vi "Harvest OAuth Test.vi"() -> ()   [LabVIEW 2013]
uses:
  Oauth2.Harvest/Harvest Access Scopes.ctl
  OauthClient/OAuthClient.lvclass
  Oauth2/Oauth2.lvclass/Oauth2.ctl
  Oauth2/Read RefreshToken.vi
  Oauth2/Read ExpiresIn.vi
  Oauth2/Read Redirect URI.vi
  OAuthToken/Retrieve Element.vi
  Oauth2/Oauth2.lvclass
  <vilib>/LabVIEW Open Source Project/OpenURI/uri/URI.lvclass
  <vilib>/httpClient/LabVIEWHTTPClient.lvlib
  Oauth2.Harvest/Oauth2.Harvest.lvclass
panel:
  in  "Access Scope":T1={"all"=TRUE, "harvest:all"=FALSE, "forercast:all"=FALSE, "harvest:{accountID}"=FALSE, "forercast:{accountID}"=FALSE}
  out "REST API Error":errorcluster
  out "HTTP Response Headers":string
  out "Accounts":string
  out "Harvest Access Token":string
  out "Refresh Token":string
  out "Expires In":u32
  out "Redirect URI":string
  in  "Harvest API URL":string="https://id.getharvest.com/api/v2"
  out "Oauth Error":errorcluster
  in  "Query API Version":bool
  in  "Refresh":bool
  in  "Authorize":bool
  in  "Client Secret":string
  in  "Client ID":string
  # "Harvest Application API Access Example"
  # "G Open Source Project for LabVIEW\nhttps://github.com/LabVIEW-Open-Source/Oauth2"
  # "1- Get a Client ID and Client Secret from the application's admin. \n\n          * To access your own account, log into your site, create an application and set the access scope. \n          * This Oauth2.0 API uses the following redirect URL: http://localhost:58888/Oauth2/Redirect\n          * Record the client ID and client secret and fill in the fields below."
  # "3- Get an Access Token. You will be redirected your Harvest App's Authorization Server URI\n              * To authorize access, click on the \"Authorize App\" button.\n\n4- Once you have authenticated yourself, you will receive an access token.\n              * Use the \"Refresh Token\" button to request a fresh token\n                       OR\n              * Use the Access Token to query the Harvest API"
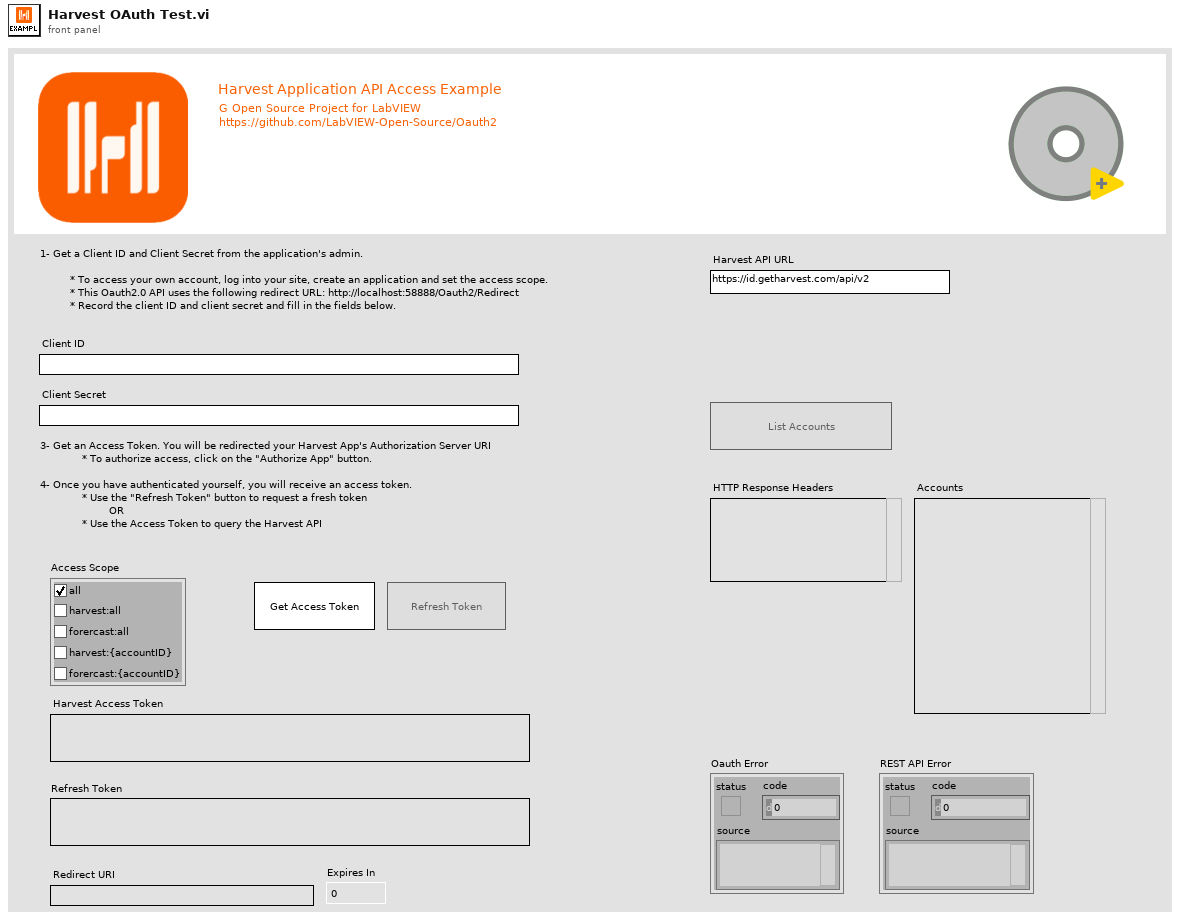
[diagram p1: front panel]
types:
  T1 = typedef "Oauth2.Harvest.lvclass/Harvest Access Scopes.ctl" = cluster{"all":bool, "harvest:all":bool, "forercast:all":bool, "harvest:{accountID}":bool, "forercast:{accountID}":bool}
  T2 = enum8{"Enabled", "Disabled", "Disabled and Grayed Out"}
  T3 = cluster{"Oauth2":refnum<class "Oauth2.Harvest.lvclass">, "Harvest API URL":string}
  T4 = typedef "LabVIEWHTTPClient.lvlib/ClientHandle.ctl" = refnum<k1>
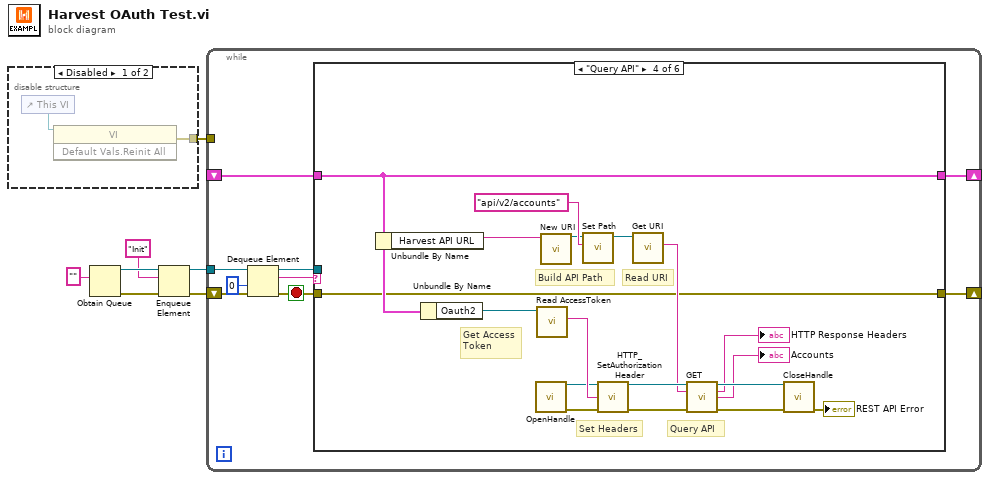
[diagram p0: block diagram]
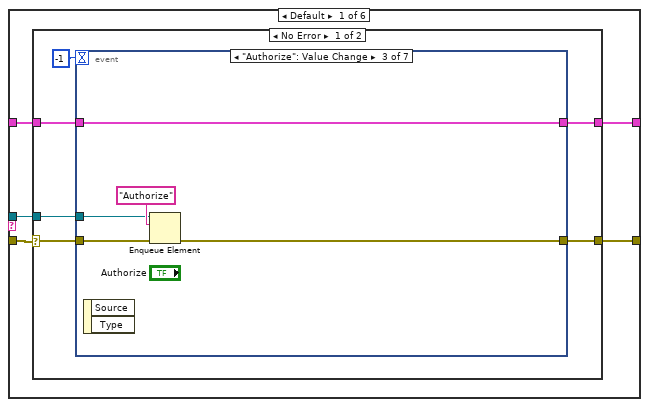
[diagram p3: hidden frame]
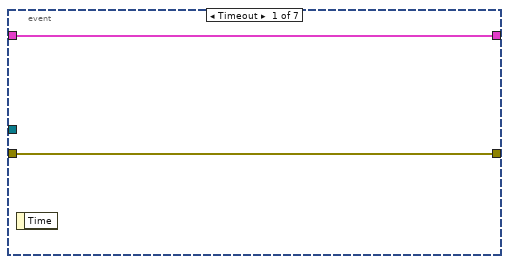
[diagram p4: hidden frame]
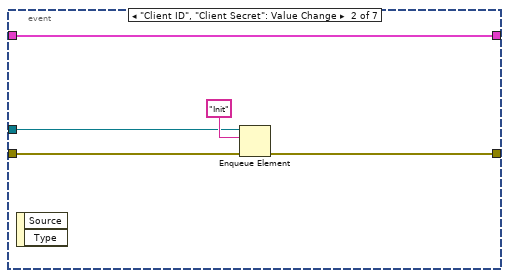
[diagram p5: hidden frame]
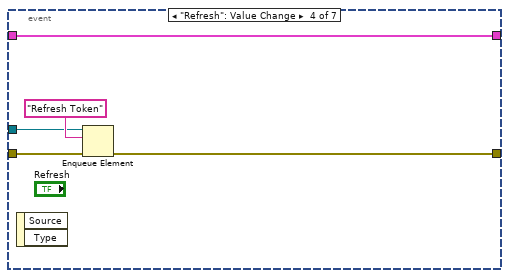
[diagram p6: hidden frame]
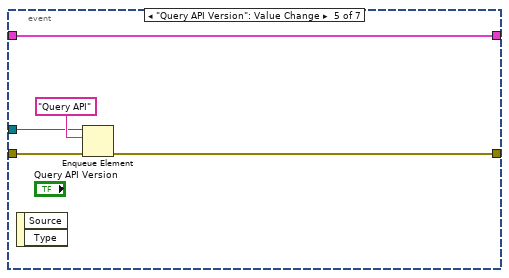
[diagram p7: hidden frame]
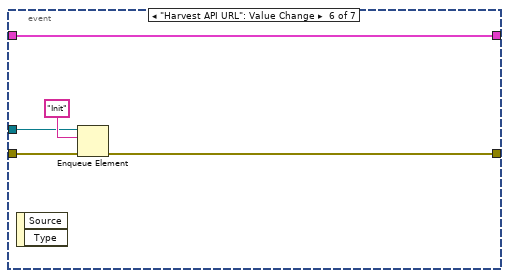
[diagram p8: hidden frame]
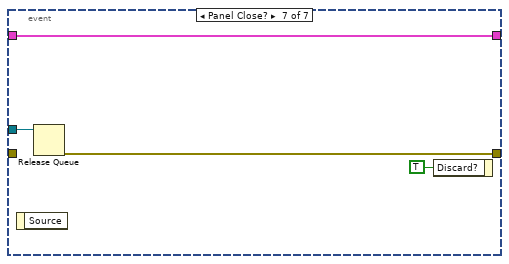
[diagram p9: hidden frame]
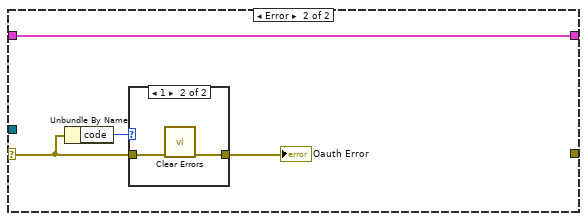
[diagram p10: hidden frame]
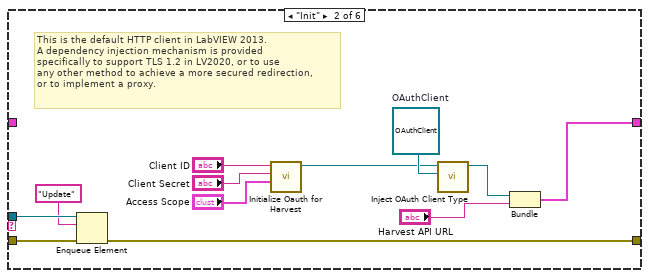
[diagram p12: hidden frame]
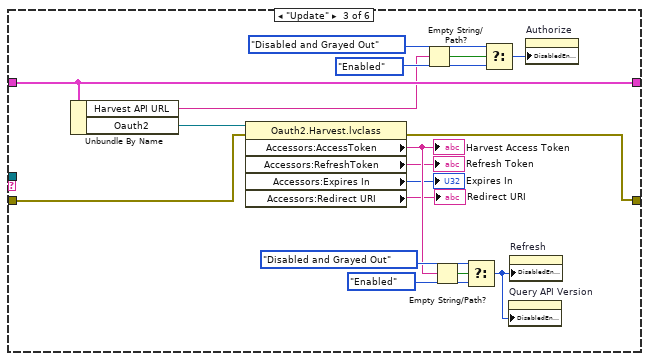
[diagram p13: hidden frame]
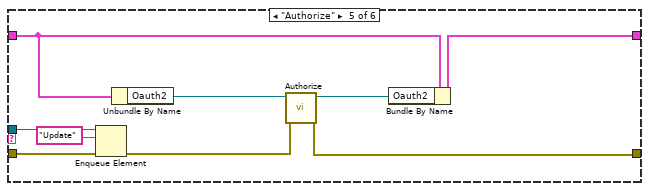
[diagram p14: hidden frame]
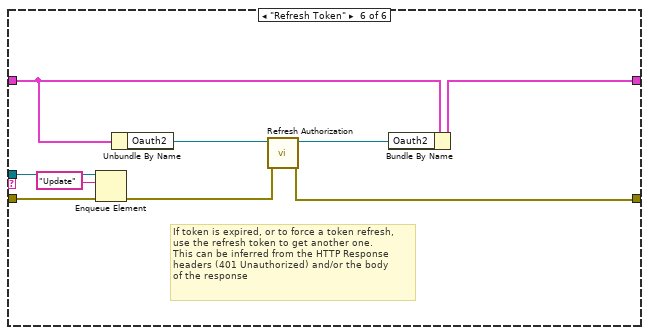
[diagram p15: hidden frame]
diagram:
  n1 = disable-structure shown="Disabled" {
    disable-tunnel: [w8 _] -> w1
    frame Disabled {
      n2 = control-ref of="This VI"() -> (w9:refnum<vi>)
      n3 = invoke class="VI" method="Default Vals.Reinit All"(reference=w9) -> (error out=w8:errorcluster)  [unwired: 2 in, 2 out]
    }
    frame Enabled {
    }
  }
  n4 = Obtain Queue(element data type="") -> (queue out=w4:refnum<queue>, error out=w6:errorcluster)  [unwired: 4 in, 1 out]
  n5 = Enqueue Element(queue=w4, element="Init", error in (no error)=w6) -> (queue out=w3:refnum<queue>, error out=w5:errorcluster)  [unwired: 1 in, 1 out]
  n6 = while {
    tunnel: w3 -> [w18]
    shift-right: [w13] -> _
    shift-left: _ -> [w12]
    shift-right: [w10] -> _
    shift-left: w5 -> [w14]
    tunnel: w1 -> [_]
    stop <- w11 stop-if-true
    n7 = Dequeue Element(queue=w18, timeout in ms (-1)=0, error in (no error)=w14) -> (queue out=w15:refnum<queue>, element=w16:string, error out=w11:errorcluster)  [unwired: 1 out]
    n8 = case shown="\"Query API\"" w16 {
      tunnel: w15 -> [w23 w78 _ _ w117 w129]
      tunnel: [w22 w79 w96 w111 w119 w131] -> w13
      tunnel: w12 -> [w21 _ w96 w111 w120 w132]
      tunnel: w11 -> [w20 w75 w86 w99 w116 w128]
      tunnel: [w19 w76 w85 w99 w122 w124] -> w10
      frame Default {
        n9 = case shown="No Error" w20 {
          selector: w20 -> [w24 w63]
          tunnel: w23 -> [w28 _]
          tunnel: [w27 w64] -> w22
          tunnel: w21 -> [w26 w64]
          tunnel: [w25 _] -> w19
          frame No Error {
            n10 = event shown="[2] \"Authorize\": Value Change" {
              selector: _ -> [_ _ _ _ _ _ _]
              dyn-events: _ -> [_ _ _ _ _ _ _]
              timeout: -1 -> [_ _ _ _ _ _ _]
              tunnel: w28 -> [_ w34 w40 w45 w50 w55 w60]
              tunnel: [w31 w36 w38 w43 w48 w53 w58] -> w27
              tunnel: w26 -> [w31 w36 w38 w43 w48 w53 w58]
              tunnel: [w30 w32 w37 w42 w47 w52 w57] -> w25
              tunnel: w24 -> [w30 w33 w39 w44 w49 w54 _]
              event Timeout {
                n11 = event-data() -> ()  [unwired: 1 in, 1 out]
              }
              event "Client ID", "Client Secret": Value Change {
                n12 = event-data() -> ()  [unwired: 1 in, 2 out]
                n13 = Enqueue Element(queue=w34, element="Init", error in (no error)=w33) -> (error out=w32:errorcluster)  [unwired: 1 in, 2 out]
              }
              event "Authorize": Value Change {
                n14 = event-data() -> ()  [unwired: 1 in, 2 out]
                n15 = Enqueue Element(queue=w40, element="Authorize", error in (no error)=w39) -> (error out=w37:errorcluster)  [unwired: 1 in, 2 out]
              }
              event "Refresh": Value Change {
                n16 = event-data() -> ()  [unwired: 1 in, 2 out]
                n17 = Enqueue Element(queue=w45, element="Refresh Token", error in (no error)=w44) -> (error out=w42:errorcluster)  [unwired: 1 in, 2 out]
              }
              event "Query API Version": Value Change {
                n18 = event-data() -> ()  [unwired: 1 in, 2 out]
                n19 = Enqueue Element(queue=w50, element="Query API", error in (no error)=w49) -> (error out=w47:errorcluster)  [unwired: 1 in, 2 out]
              }
              event "Harvest API URL": Value Change {
                n20 = event-data() -> ()  [unwired: 1 in, 2 out]
                n21 = Enqueue Element(queue=w55, element="Init", error in (no error)=w54) -> (error out=w52:errorcluster)  [unwired: 1 in, 2 out]
              }
              event Panel Close? {
                n22 = event-data() -> ()  [unwired: 1 in, 1 out]
                n23 = Release Queue(queue=w60) -> (error out=w57:errorcluster)  [unwired: 2 in, 2 out]
                n24 = event-data("Discard?"=TRUE) -> ()  [unwired: 1 in, 1 out]
              }
            }
          }
          frame Error {
            n25 = Unbundle By Name(w63) -> ("code"=w61:i32)
            n26 = case shown="1" w61 {
              tunnel: w63 -> [w65 w67]
              tunnel: [w65 w66] -> w62
              frame Default {
              }
              frame 1 {
                n27 = call <vilib>:"Clear Errors.vi"("error in (no error)"=w67) -> ("error out"=w66:errorcluster)  [unwired: 6 in]
              }
            }
            "Oauth Error" <- w62
          }
        }
      }
      frame "Init" {
        w74 = refnum<class "OAuthClient.lvclass"> refnum  # OAuthClient
        # "This is the default HTTP client in LabVIEW 2013.\nA dependency injection mechanism is provided\nspecifically to support TLS 1.2 in LV2020, or to use\nany other method to achieve a more secured redirection, \nor to implement a proxy."
        n28 = Enqueue Element(queue=w78, element="Update", error in (no error)=w75) -> (error out=w76:errorcluster)  [unwired: 1 in, 2 out]
        n29 = call "Initialize Oauth for Harvest.vi"("Harvest Access Scope"="Access Scope", "Client Secret"="Client Secret", "Client ID"="Client ID") -> ("Oauth2.Harvest"=w69:refnum<class "Oauth2.Harvest.lvclass">)  [unwired: 7 in, 1 out]
        n30 = call "Inject OAuth Client Type.vi"("OAuthClient"=w74, "Oauth2 in"=w69) -> ("Oauth2"=w73:refnum<class "Oauth2.Harvest.lvclass">)  [unwired: 9 in]
        n31 = Bundle("Oauth2"=w73, "Harvest API URL"="Harvest API URL") -> (w79:T3)  [unwired: 1 in]
      }
      frame "Update" {
        n32 = Unbundle By Name(w96) -> ("Harvest API URL"=w90:string, "Oauth2"=w91:refnum<class "Oauth2.Harvest.lvclass">)
        n33 = property class="Oauth2.Harvest.lvclass"(reference=w91, error in=w86) -> (error out=w85:errorcluster, "Accessors:AccessToken"=w84:string, "Accessors:RefreshToken"=→"Refresh Token":string, "Accessors:Expires In"=→"Expires In":u32, "Accessors:Redirect URI"=→"Redirect URI":string)  [unwired: 1 out]
        "Harvest Access Token" <- w84
        n34 = Empty String/Path?(string/path=w90) -> (empty?=w93:bool)
        n35 = Empty String/Path?(string/path=w84) -> (empty?=w89:bool)
        n36 = Select(t=T2."Disabled and Grayed Out" ("Disabled"), s=w89, f=T2."Enabled" ("Disabled")) -> (s? t:f=w80:T2)
        n37 = Select(t=T2."Disabled and Grayed Out" ("Disabled"), s=w93, f=T2."Enabled" ("Disabled")) -> (s? t:f=w92:T2)
        n38 = property on="Query API Version" class="Bool"("DisabledEnum"=w80) -> ()  [unwired: 2 in, 2 out]
        n39 = property on="Refresh" class="Bool"("DisabledEnum"=w80) -> ()  [unwired: 2 in, 2 out]
        n40 = property on="Authorize" class="Bool"("DisabledEnum"=w92) -> ()  [unwired: 2 in, 2 out]
      }
      frame "Query API" {
        # "Query API"
        # "Set Headers"
        # "Get Access\nToken"
        # "Read URI"
        # "Build API Path"
        n41 = Unbundle By Name(w111) -> ("Harvest API URL"=w107:string)
        n42 = Unbundle By Name(w111) -> ("Oauth2"=w112:refnum<class "Oauth2.Harvest.lvclass">)
        n43 = call <vilib>:"OpenHandle.vi"() -> ("client handle out"=w113:T4, "error out"=w104:errorcluster)  [unwired: 14 in]
        n44 = call "Read AccessToken.vi"("Oauth2 in"=w112) -> ("Access Token"=w114:string)  [unwired: 8 in, 2 out]
        n45 = call <vilib>:"New URI.vi"("URI"=w107) -> ("URI"=w108:refnum<class "URI.lvclass">)  [unwired: 9 in, 1 out]
        n46 = call <vilib>:"Set Path.vi"("path"="api/v2/accounts", "URI in"=w108) -> ("URI out"=w110:refnum<class "URI.lvclass">)  [unwired: 8 in, 1 out]
        n47 = call "HTTP_SetAuthorizationHeader.vi"("Client Handle"=w113, "Access Token"=w114, "error in (no error)"=w104) -> ("client handle dup"=w106:T4, "error out"=w103:errorcluster)  [unwired: 11 in]
        n48 = call <vilib>:"Get URI.vi"("URI in"=w110) -> ("URI String"=w105:string)  [unwired: 8 in, 2 out]
        n49 = call <vilib>:"GET.vi"("client handle"=w106, "url"=w105, "error in (no error)"=w103) -> ("client handle out"=w102:T4, "headers"=→"HTTP Response Headers":string, "body"=→"Accounts":string, "error out"=w101:errorcluster)  [unwired: 9 in]
        n50 = call <vilib>:"CloseHandle.vi"("client handle"=w102, "error in (no error)"=w101) -> ("error out"=→"REST API Error":errorcluster)  [unwired: 13 in]
      }
      frame "Authorize" {
        n51 = Enqueue Element(queue=w117, element="Update", error in (no error)=w116) -> (error out=w115:errorcluster)  [unwired: 1 in, 2 out]
        n52 = Unbundle By Name(w120) -> ("Oauth2"=w123:refnum<class "Oauth2.Harvest.lvclass">)
        n53 = call "Authorize.vi"("error in (no error)"=w115, "Oauth2 in"=w123) -> ("error out"=w122:errorcluster, "Oauth2 out"=w121:refnum<class "Oauth2.Harvest.lvclass">)  [unwired: 7 in, 1 out]
        n54 = Bundle By Name(cluster=w120, "Oauth2"=w121) -> (w119:T3)
      }
      frame "Refresh Token" {
        # "If token is expired, or to force a token refresh, \nuse the refresh token to get another one.\nThis can be inferred from the HTTP Response\nheaders (401 Unauthorized) and/or the body\nof the response"
        n55 = Enqueue Element(queue=w129, element="Update", error in (no error)=w128) -> (error out=w125:errorcluster)  [unwired: 1 in, 2 out]
        n56 = Unbundle By Name(w132) -> ("Oauth2"=w127:refnum<class "Oauth2.Harvest.lvclass">)
        n57 = call "Refresh Authorization.vi"("error in (no error)"=w125, "Oauth2 in"=w127) -> ("error out"=w124:errorcluster, "Oauth2 out"=w126:refnum<class "Oauth2.Harvest.lvclass">)  [unwired: 7 in, 1 out]
        n58 = Bundle By Name(cluster=w132, "Oauth2"=w126) -> (w131:T3)
      }
    }
  }
